vi "PTScanner.set i attribute.vi"(0 "i ref in":refnum<vi>, 2 "i attribute":T1, 5 "error in (no error)":errorcluster) -> (14 "i ref out":refnum<vi>, 19 "error out":errorcluster)   [LabVIEW 2014, in "PTScanner.lvlib"]
uses:
  PTScanner.lvlib
  PTScanner.i attribute.ctl
  PTScanner.obj parameters.ctl
  PTScanner.step obj parameters.ctl
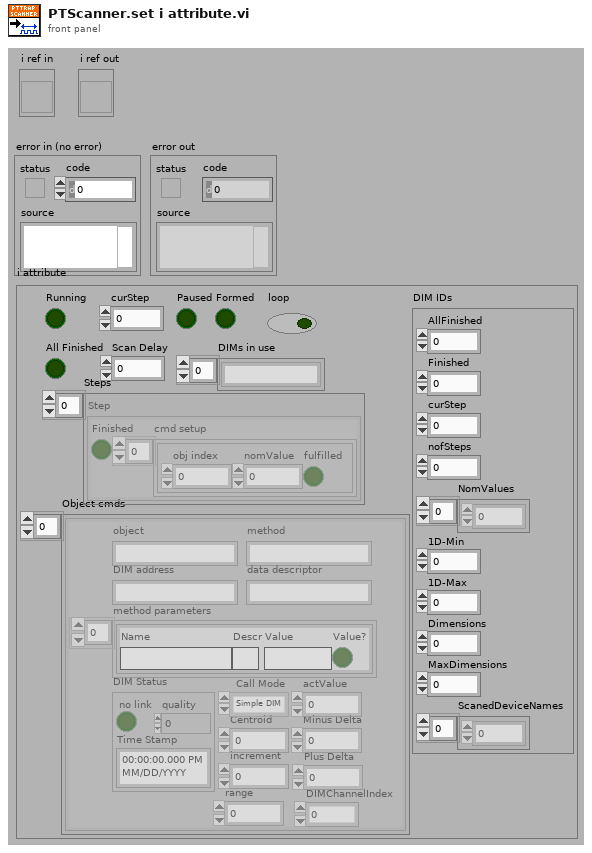
[diagram p1: front panel]
types:
  T1 = typedef "PTScanner.lvlib/PTScanner.i attribute.ctl" = cluster{"Object cmds":T2[], "Steps":cluster{"Finished":bool, "cmd setup":T3[]}[], "curStep":i32, "DIM IDs":cluster{"AllFinished":i32, "Finished":i32, "curStep":i32, "nofSteps":i32, "NomValues":i32[], "1D-Min":i32, "1D-Max":i32, "Dimensions":i32, "MaxDimensions":i32, "ScanedDeviceNames":i32[]}, "All Finished":bool, "DIMs in use":string[], "Running":bool, "Scan Delay":u32, "loop":bool, "Paused":bool, "Formed":bool}
  T2 = typedef "PTScanner.lvlib/PTScanner.obj parameters.ctl" = cluster{"object":string, "DIM address":string, "method":string, "data descriptor":string, "method parameters":cluster{"Name":string, "Descr":string, "Value":string, "Value?":bool}[], "Call Mode":enum16{"Simple DIM", "Synchronous"}, "actValue":dbl, "Centroid":dbl, "Minus Delta":dbl, "Plus Delta":dbl, "increment":dbl, "DIM Status":cluster{"no link":bool, "quality":i32, "Time Stamp":timestamp}, "range":dbl, "DIMChannelIndex":i32}
  T3 = typedef "PTScanner.lvlib/PTScanner.step obj parameters.ctl" = cluster{"obj index":i32, "nomValue":dbl, "fulfilled":bool}
  T4 = enum16{"SetAttribute", "GetAttribute", "CreateAttribute", "DestroyAttribute", "DestroyAllAtributes"}
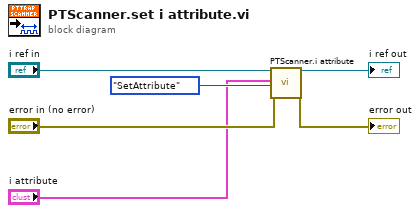
[diagram p0: block diagram]
diagram:
  n1 = call "PTScanner.i attribute.vi"("VI Refnum"="i ref in", "CLASS.i attribute"="i attribute", "Action"=T4."SetAttribute", "error in (no error)"="error in (no error)") -> ("VI Refnum out"=→"i ref out":refnum<vi>, "error out"=→"error out":errorcluster)  [unwired: 13 in, 1 out]
